vi "Dashboard Main Old.vi"() -> ()   [LabVIEW 2020]
uses:
  <vilib>/Rock Robotics/Network Tables/NT Read Numeric Array.vi
  <vilib>/Rock Robotics/Network Tables/NT Read String.vi
  <vilib>/Rock Robotics/Network Tables/NT Read Number.vi
  <vilib>/Rock Robotics/Network Tables/NT Read Boolean.vi
  <vilib>/Rock Robotics/Network Tables/NT Write Number.vi
  <vilib>/Rock Robotics/Network Tables/NT Write Boolean.vi
panel:
  out "Popcorn Engaged":bool
  out "Camera Image 5":T1(plugin-control)
  in  "Camera Settings Right":T2={"Frame Rate"=30, "Compression"=30, "Size"=1, "DB Camera Config"=FALSE} {"Frame Rate" scale=1.0..30.0; "Compression" scale=100.0..-1.0; "Size" items=["640x480", "320x240", "160x120"]}
  in  "Camera Name Right":string(combo)="No Camera Selection"
  out "Camera Perf":string
  in  "Camera Settings":T2={"Frame Rate"=30, "Compression"=30, "Size"=1, "DB Camera Config"=FALSE} {"Frame Rate" scale=1.0..30.0; "Compression" scale=100.0..-1.0; "Size" items=["640x480", "320x240", "160x120"]}
  in  "TCP":refnum<k5>
  out "Robot IP":string
  in  "Dashboard Tab":T3(tab)
  out "MotorChart R":cluster{"Numeric":dbl, "Numeric":dbl}(graph)
  out "MotorChart L":cluster{"Numeric":dbl, "Numeric":dbl}(graph)
  out "MotorSliders R":cluster{"MotorSlide1":dbl, "MotorSlide2":dbl} {"MotorSlide2" scale=-1.0..1.0 scale format="%#_2e"; "MotorSlide1" scale=-1.0..1.0 scale format="%#_2e"}
  out "MotorSliders L":cluster{"MotorSlide1":dbl, "MotorSlide2":dbl} {"MotorSlide2" scale=-1.0..1.0 scale format="%#_2e"; "MotorSlide1" scale=-1.0..1.0 scale format="%#_2e"}
  out "To infinity and beyond?":string
  out "Climb Override":bool
  out "Climbing Stages":sgl(slide) scale=0.0..10.0 scale format="%#_6p"
  out "Reverse":bool
  in  "ARE YOU READY TO RUMBLE":bool
  out "Drive Mode":string
  in  "Select Auto":string(combo)="Select Autonomous ..."
  out "NT Connection":bool
  out "JS1 Z":dbl(slide) scale=-1.0..1.0 scale format="%#_2e"
  out "JS1 Graph":cluster{"X":dbl, "Y":dbl}[](graph)
  out "JS1 Buttons":T4
  out "JS2 Z":dbl(slide) scale=-1.0..1.0 scale format="%#_2e"
  out "JS2 Graph":cluster{"X":dbl, "Y":dbl}[](graph)
  out "JS2 Buttons":T4
  out "Lidar":dbl(knob) scale=0.0..10.0
  out "Wall!":bool
  out "Mode":T5(ring)=enum."Auto Disabled"
  out "Camera Image Right":T1(plugin-control)
  out "Shooter Speed":cluster{"Shooter Demand":dbl, "Numeric":dbl}(graph)
  out "Shooter Speed":dbl
  in  "Shooter Demand":dbl
  in  "Dashboard Tab 2":T6(tab)
  out "Speed Chart Left":cluster{"Numeric":dbl, "Numeric":dbl}(graph)
  out "Speed Chart Right":cluster{"Numeric":dbl, "Numeric":dbl}(graph)
  in  "Boolean":bool
  out "Right Speed Demand":dbl
  out "Left Speed Demand":dbl
  out "Right Speed":dbl
  out "Left Speed":dbl
  out "Current Filter":T7={"Hue"={110.0, 142.0}, "Saturation"={0.0, 209.6394230769231}, "Value"={0.0, 105.16949152542372}} {"Value" scale=0.0..255.0; "Saturation" scale=0.0..255.0; "Hue" scale=0.0..255.0 scale format="%#_3g"}
  in  "New Filter":T7={"Hue"={110.0, 142.0}, "Saturation"={0.0, 209.6394230769231}, "Value"={0.0, 105.16949152542372}} {"Value" scale=0.0..255.0; "Saturation" scale=0.0..255.0; "Hue" scale=0.0..255.0 scale format="%#_3g"}
  out "Bananas Engaged":bool
  in  "DONUT PRESS":bool
  out "Bandwidth (Mbps)":dbl
  out "FPS":dbl
  in  "Update":bool
  in  "CheckList":i32[](listbox)
  out "Tree":string(tree)
  out "Camera Image":T1(plugin-control)
  out "Background":bool
  in  "Camera Name":string(combo)="No Camera Selection"
  # "HW"
  # "HW"
  # "Drive Motors"
  # "Joysticks"
  # "Front"
  # "Right"
  # "Left"
  # "Back"
  # "Right"
  # "Left"
  # "Speed D"
  # "Speed"
  # "DONUT PRESS"
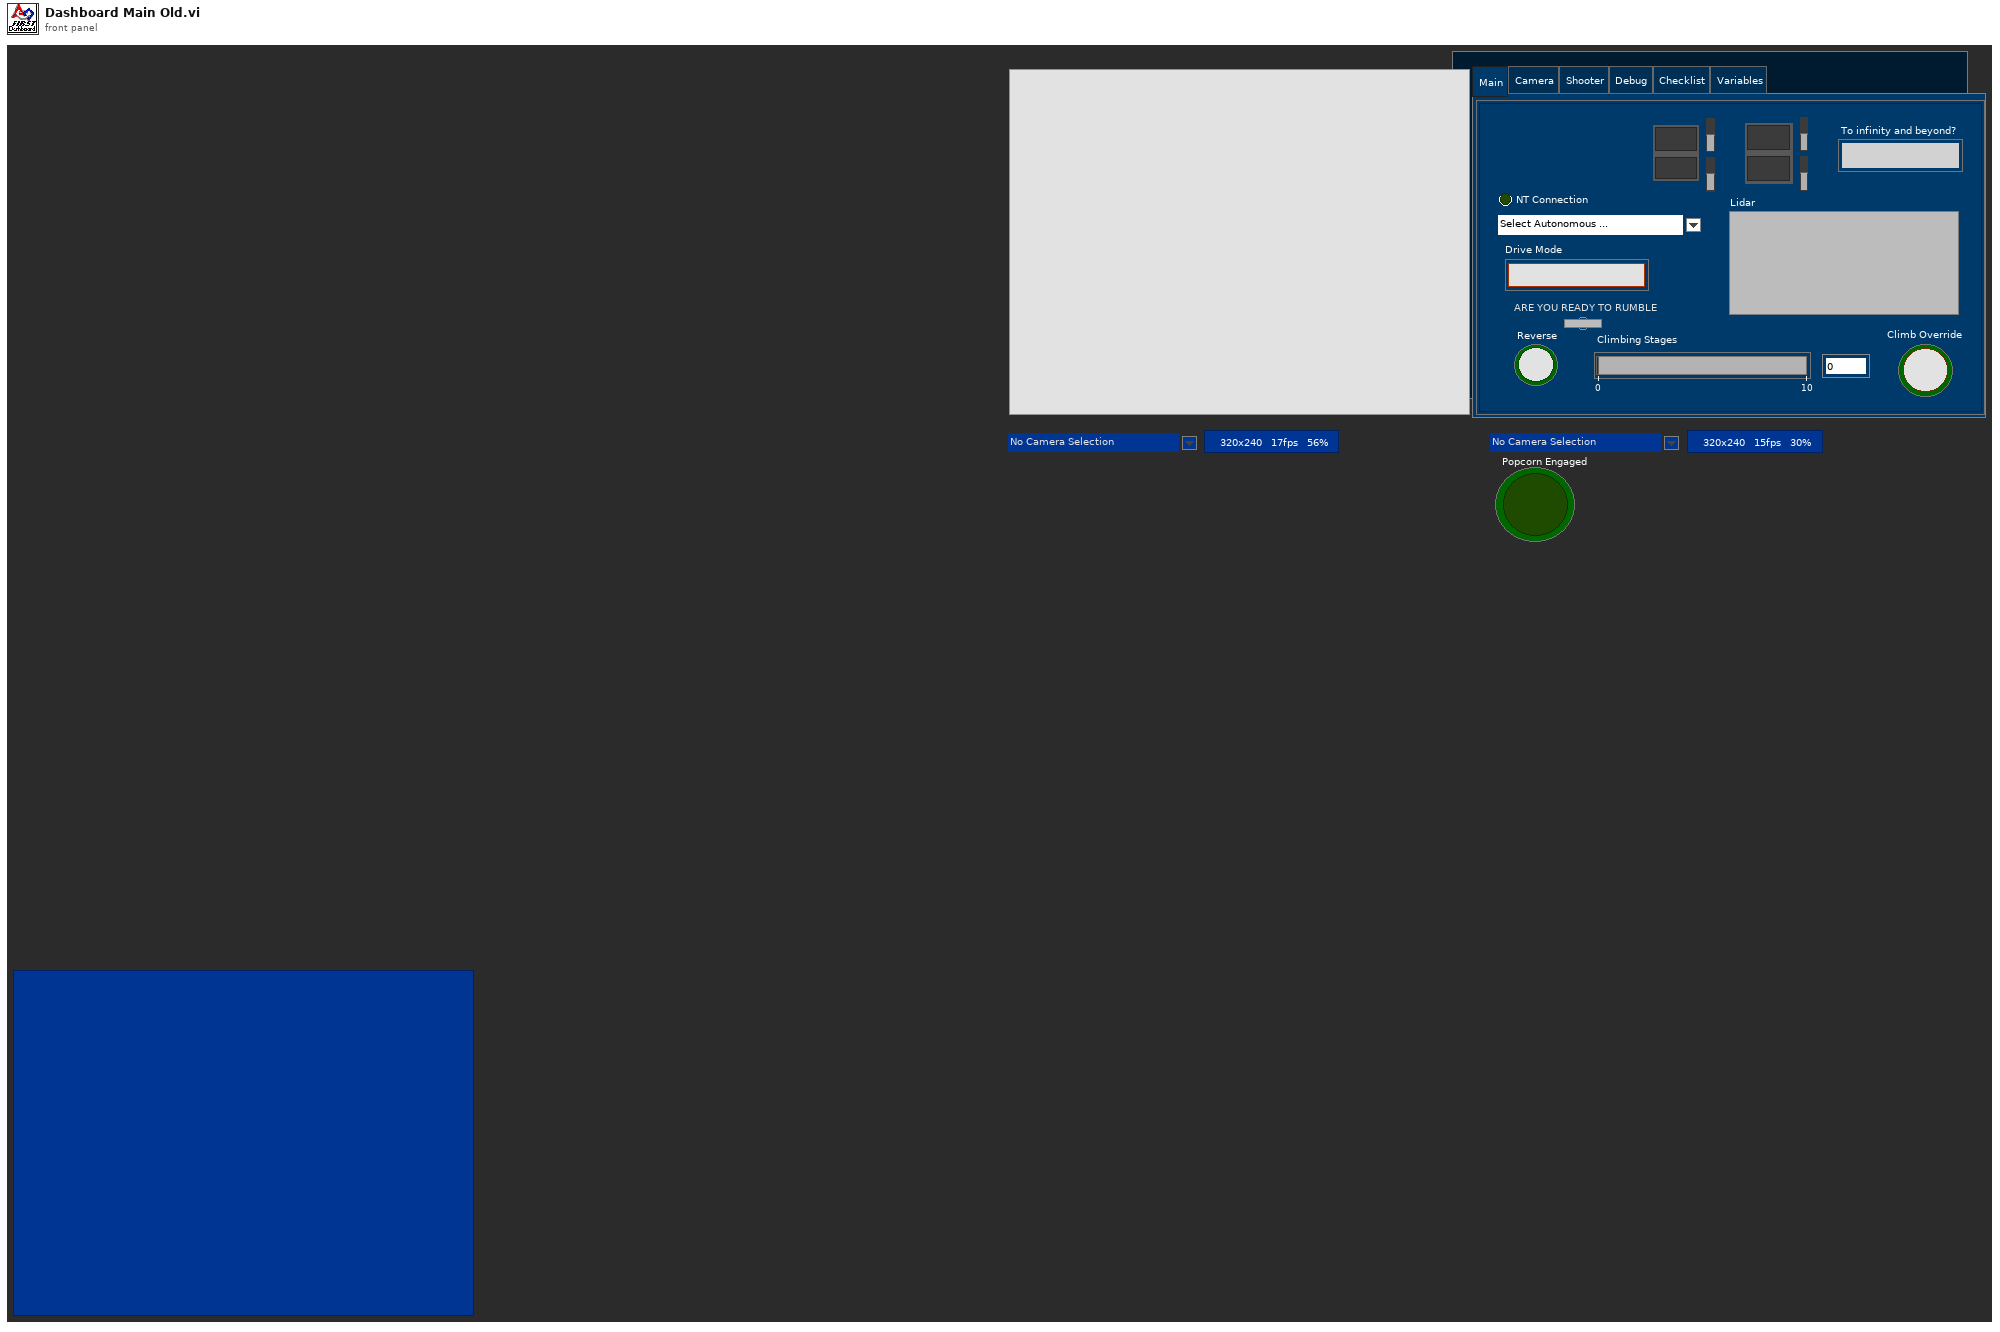
[diagram p1: front panel]
types:
  T1 = typedef "IMAQ Image.ctl" = refnum<image>
  T2 = cluster{"Frame Rate":i32, "Compression":i32, "Size":u16, "DB Camera Config":bool}
  T3 = enum32{"Main", "Camera", "Shooter", "Debug", "Checklist", "Variables"}
  T4 = cluster{bool, bool, bool, bool, bool, bool, bool, bool, bool, bool, bool, bool}
  T5 = enum8{"Tele-Op Disabled", "Tele-Op Enabled", "Auto Disabled", "Auto Enabled", "Test Disabled", "Test Enabled", "Disconnected", "No Code", "E-Stop"}
  T6 = enum32{"Drive Left", "Drive Right", "Table", "Camera", "Random"}
  T7 = cluster{"Hue":cluster{dbl, dbl}, "Saturation":cluster{dbl, dbl}, "Value":cluster{dbl, dbl}}
  T8 = typedef "Image Type" = u32
  T9 = cluster{"Save Path":path, "Interval (s)":dbl, "Keep":i32}
  T10 = cluster{"Camera Image":refnum<vi>, "Dashboard Tab":refnum<vi>, "Background":refnum<vi>, "Tree":refnum<vi>, "Camera Settings":refnum<vi>, "Camera Name":refnum<vi>, "Camera Perf":refnum<vi>}
  T11 = cluster{"Camera Name":string, "Camera File Name":string, "Saved DB Images Info":cluster{"Save Path":path, "Interval (s)":dbl, "Keep":i32}}
  T12 = cluster{cluster{dbl, dbl}, cluster{dbl, dbl}, cluster{dbl, dbl}}
  T13 = cluster{"Shift":bool, "Ctrl":bool, "Alt":bool, "Cmd":bool, "Opt":bool}
  T14 = cluster{"Global Rectangle":i32[], "Contours":cluster{"Contour Type":u32, "ROI Type":u32, "Points":i32[]}[]}
  T15 = cluster{"Camera Name Right":string, string, "Saved DB Images Info":cluster{"Save Path":path, "Interval (s)":dbl, "Keep":i32}}
  T16 = cluster{"Error Strings":string, "Disable Counts":cluster{u16, u16}, "Rail Faults":cluster{u16, u16, u16}, "Robot IP":string, "DB Mode":u8, "Event Info":cluster{"Name":string, "Type":u8, "Number":u16, "Replay":u8}}
  T17 = cluster{"Storage":cluster{"Disk Free":u64, "RAM Block":u32, "RAM free":u32}, "CPU Utilization":cluster{"CPU % ISR":sgl, "CPU % Time Crit":sgl, "CPU % Timed Str":sgl, "CPU % High":sgl, "CPU % Above":sgl, "CPU % Normal":sgl, "CPU % Low":sgl}, "CAN":cluster{"% Bus Utilization":sgl, "Bus Off Cnt":u32, "TX_FIFO Full Cnt":u32, "Receive Error Cnt":u8, "Transmit Error Cnt":u8}, "HID":cluster{"HID Outputs":u32, "Rumble Low":u16, "Rumble High":u16}[]}
  T18 = cluster{"Status bits":cluster{"Test Mode":bool, "Autonomous":bool, "Enabled":bool, "Code Start":bool, "Brownout":bool, "Reserved 2":bool, "Reserved 3":bool, "E-Stop":bool}, "Code Trace":cluster{"Disabled":bool, "TeleOp":bool, "Auto":bool, "Test":bool}, "Controller Type":enum16{"unknown", "cRIO", "roboRio"}, "Code?":enum16{"unknown", "noCode", "code"}, "Battery V":dbl}
  T19 = cluster{"Control Bits":cluster{"TestMode":bool, "Autonomous":bool, "Enabled":bool, "FMS Present":bool, bool, bool, bool, "E-Stop":bool}, "Team Station ":u8, "Countdown":sgl, "Joystick Values":cluster{"Axes":dbl[], "Buttons":bool[], "POVs":i16[]}[]}
  T20 = cluster{"Axes":dbl[], "Buttons":bool[], "POVs":i16[]}[]
  T21 = cluster{"Axes":dbl[], "Buttons":bool[], "POVs":i16[]}
  T22 = cluster{"Buttons[0]":bool, "Buttons[1]":bool, "Buttons[2]":bool, "Buttons[3]":bool, "Buttons[4]":bool, "Buttons[5]":bool, "Buttons[6]":bool, "Buttons[7]":bool, "Buttons[8]":bool, "Buttons[9]":bool, "Buttons[10]":bool, "Buttons[11]":bool}
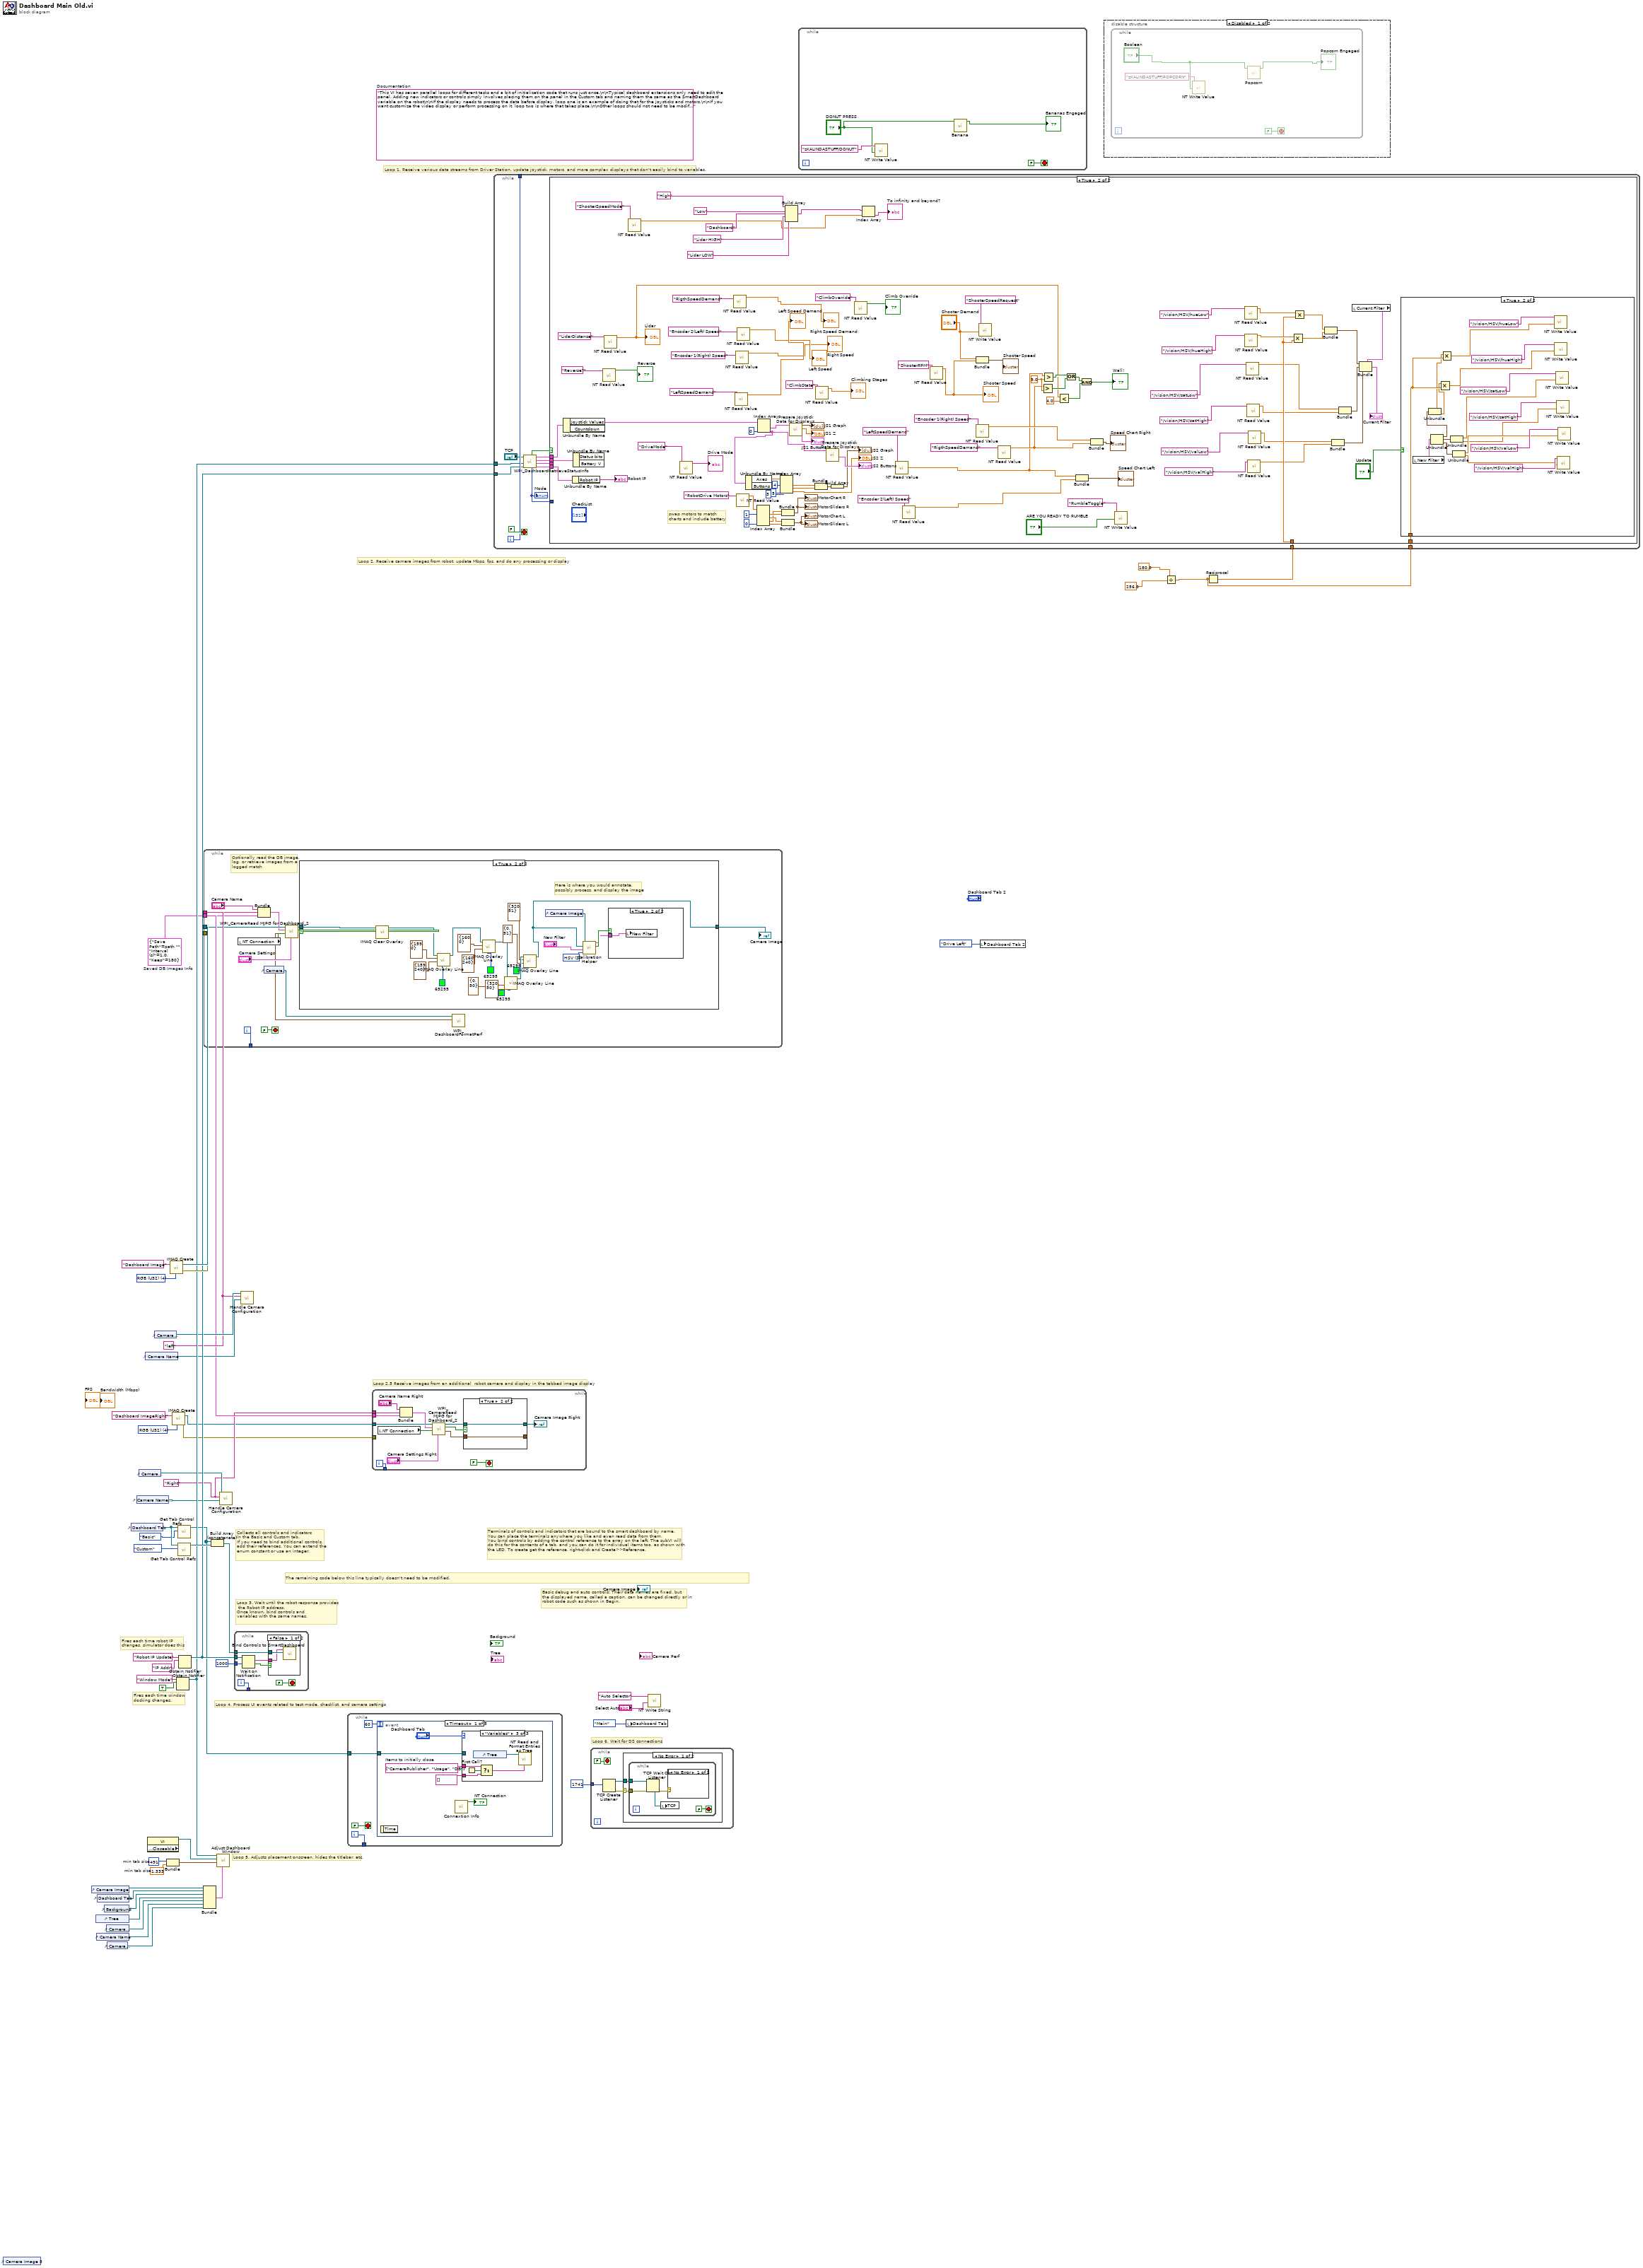
[diagram p0: block diagram]
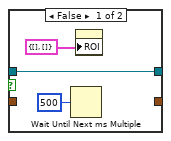
[diagram p3: hidden frame]
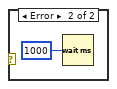
[diagram p4: hidden frame]
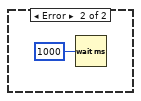
[diagram p5: hidden frame]
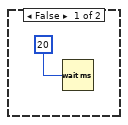
[diagram p6: hidden frame]
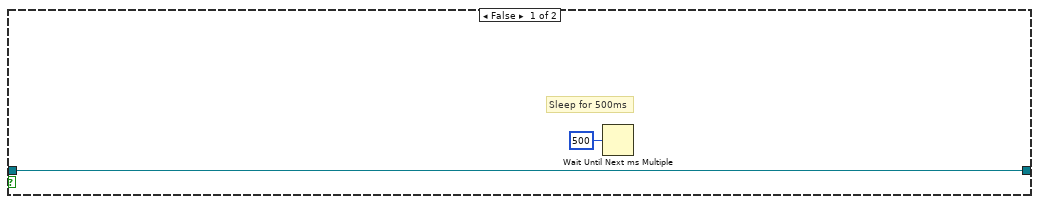
[diagram p9: hidden frame]
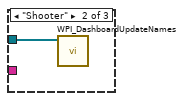
[diagram p12: hidden frame]
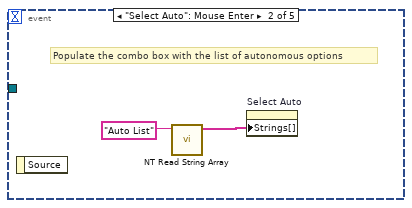
[diagram p13: hidden frame]
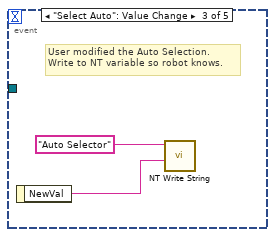
[diagram p14: hidden frame]
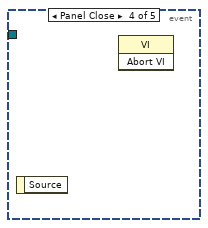
[diagram p15: hidden frame]
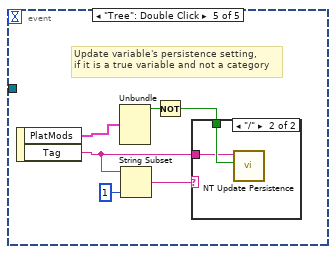
[diagram p16: hidden frame]
diagram:
  w8 = T8 4 items=["Grayscale (U8)", "Grayscale (I16)", "Grayscale (SGL)", "Complex (CSG)", "RGB (U32)", "HSL (U32)", "RGB (U64)"] ("Image Type")
  w10 = "Right"
  w14 = "left" ("Camera File Name")
  w13 = T9 {"Save Path"=path "", "Interval (s)"=1.0, "Keep"=180}  # Saved DB Images Info
  w34 = 491  # min tab size
  w33 = 1.333  # min tab size
  (unwired) "This VI has seven parallel loops for different tasks and a bit of initialization code that runs just once.\n\nTypical dashboard extensions only need to edit the panel. Adding new indicators or controls simply involves placing them on the panel in the Custom tab and naming them the same as the SmartDashboard variable on the robot\n\nIf the display needs to process the data before display, loop one is an example of doing that for the joysticks and motors.\n\nIf you want customize the video display or perform processing on it, loop two is where that takes place.\n\nOther loops should not need to be modified. They are pretty standard, and document the task they perform."  # Documentation
  w49 = T8 4 items=["Grayscale (U8)", "Grayscale (I16)", "Grayscale (SGL)", "Complex (CSG)", "RGB (U32)", "HSL (U32)", "RGB (U64)"] ("Image Type")
  # "Loop 2.5 Receive images from an additional  robot camera and display in the tabbed image display"
  # "Loop 6. Wait for DS connections"
  # "Basic debug and auto controls: Their data names are fixed, but\nthe displayed name, called a caption, can be changed directly or in\nrobot code such as shown in Begin."
  # "Fires each time robot IP\nchanges, simulator does this"
  # "Fires each time window\ndocking changes."
  # "Collects all controls and indicators\nin the Basic and Custom tab.\nIf you need to bind additional controls,\nadd their references. You can extend the\nenum constant or use an integer."
  # "The remaining code below this line typically doesn't need to be modified."
  # "Loop 4. Process UI events related to test mode, checklist, and camera settings"
  # "Terminals of controls and indicators that are bound to the smart dashboard by name.\nYou can place the terminals anywhere you like and even read data from them.\nYou bind controls by adding the control reference to the array on the left. The subVI will\ndo this for the contents of a tab, and you can do it for individual items too, as shown with\nthe LED. To create get the reference, right-click and Create>>Reference."
  # "Loop 3. Wait until the robot response provides\n the Robot IP address.\nOnce known, bind controls and\nvariables with the same names."
  # "Loop 5. Adjusts placement onscreen, hides the titlebar, etc."
  # "Loop 1. Receive various data streams from Driver Station, update joystick, motors, and more complex displays that don't easily bind to variables."
  # "Loop 2. Receive camera images from robot, update Mbps, fps, and do any processing or display"
  n1 = control-ref of="Camera Image 5"() -> ()  [unwired: 1 out]
  n2 = control-ref of="Camera Image"() -> (w36:refnum<vi>)
  n3 = control-ref of="Tree"() -> (w20:refnum<vi>)
  n4 = control-ref of="Camera Name"() -> (w18:refnum<vi>)
  n5 = control-ref of="Dashboard Tab"() -> (w35:refnum<vi>)
  n6 = control-ref of="Background"() -> (w31:refnum<vi>)
  n7 = control-ref of="Camera Settings"() -> (w19:refnum<vi>)
  n8 = control-ref of="Camera Perf"() -> (w17:refnum<vi>)
  n9 = control-ref of="Dashboard Tab"() -> (w39:refnum<vi>)
  n10 = control-ref of="Camera Name Right"() -> (w11:refnum<vi>)
  n11 = control-ref of="Camera Settings Right"() -> (w12:refnum<vi>)
  n12 = control-ref of="Camera Name"() -> (w24:refnum<vi>)
  n13 = property class="VI" props=["Front Panel.Closeable"]() -> (reference out=w40:refnum<vi>)  [unwired: 2 in, 2 out]
  n14 = control-ref of="Camera Settings"() -> (w25:refnum<vi>)
  n15 = Bundle("min tab size"=w34, "min tab size"=w33) -> (w32:cluster{"min tab size":i32, "min tab size":dbl})  [unwired: 1 in]
  n16 = call "IMAQ Create"("Image Name"="Dashboard Image", "Image Type"=w49) -> ("New Image"=w47:T1, "error out"=w46:errorcluster)  [unwired: 2 in, 1 out]
  n17 = call "IMAQ Create"("Image Name"="Dashboard ImageRight", "Image Type"=w8) -> ("New Image"=w7:T1, "error out"=w6:errorcluster)  [unwired: 2 in, 1 out]
  n18 = Obtain Notifier(name (unnamed)="Window Mode", notification data type=TRUE) -> (notifier out=w28:refnum<notifier>)  [unwired: 2 in, 2 out]
  n19 = call <vilib>:"Get Tab Control Refs.vi"("Page Index"=enum32{"Drive", "Basic", "Custom", "Variables"}."Basic" ("Dashboard Tab"), "TabControl in"=w39) -> ("ControlsOnPage"=w23:refnum<vi>[])  [unwired: 9 in]
  n20 = call <vilib>:"Get Tab Control Refs.vi"("Page Index"=enum32{"Drive", "Basic", "Custom", "Variables"}."Custom" ("Dashboard Tab"), "TabControl in"=w39) -> ("ControlsOnPage"=w38:refnum<vi>[])  [unwired: 9 in]
  n21 = Obtain Notifier(name (unnamed)="Robot IP Update", notification data type="IP Addr" ("name (unnamed)")) -> (notifier out=w29:refnum<notifier>)  [unwired: 2 in, 2 out]
  n22 = Bundle("Camera Image"=w36, "Dashboard Tab"=w35, "Background"=w31, "Tree"=w20, "Camera Settings"=w19, "Camera Name"=w18, "Camera Perf"=w17) -> (w30:T10)  [unwired: 1 in]
  n23 = while {
    tunnel: w47 -> [w61]
    tunnel: w46 -> [_]
    tunnel: [w62] -> _
    tunnel: w13 -> [w55]
    tunnel: w14 -> [w53]
    i -> [w62]
    stop <- FALSE stop-if-true
    # "Optionally read the DB image,\nlog, or retrieve images from a\nlogged match"
    n24 = local read "NT Connection"() -> (w56:bool)
    n25 = Bundle("Camera Name"="Camera Name", "Camera File Name"=w53, "Saved DB Images Info"=w55) -> (w54:T11)  [unwired: 1 in]
    n26 = control-ref of="Camera Perf"() -> (w51:refnum<vi>)
    n27 = call <vilib>:"WPI_CameraRead MJPG for Dashboard_2.vi"("Camera Settings"="Camera Settings", "NT Connection"=w56, "Capture Info"=w54, "Image in"=w61) -> ("perf info"=w52:cluster{"Bandwidth (Mbps)":dbl, "fps":dbl}, "Active"=w59:bool, "Image\\ out"=w60:T1)  [unwired: 5 in]
    n28 = case shown="True" w59 {
      tunnel: w60 -> [w64 w88]
      tunnel: [w64 w72] -> w57
      frame False {
        # "Sleep for 500ms"
        n29 = Wait Until Next ms Multiple(millisecond multiple=u32 500) -> ()  [unwired: 1 out]
      }
      frame True {
        w84 = u16 2 items=["RGB", "HSL", "HSV", "HSI", "CIE L*a*b*", "CIE XYZ"] ("Color Mode")
        # "Here is where you would annotate,\npossibly process, and display the image"
        n30 = call "IMAQ Clear Overlay"("Image"=w88) -> ("Image Out"=w82:T1)  [unwired: 2 in, 8 out]
        n31 = call "IMAQ Overlay Line"("Color"=u32 65295, "End Point"=cluster{"X":i32, "Y":i32} {"X"=159, "Y"=240}, "Start Point"=cluster{"X":i32, "Y":i32} {"X"=159, "Y"=0}, "Image"=w82) -> ("Image Out"=w78:T1)  [unwired: 6 in, 1 out]
        n32 = call "IMAQ Overlay Line"("Color"=u32 65295, "End Point"=cluster{"X":i32, "Y":i32} {"X"=160, "Y"=240}, "Start Point"=cluster{"X":i32, "Y":i32} {"X"=160, "Y"=0}, "Image"=w78) -> ("Image Out"=w73:T1)  [unwired: 6 in, 1 out]
        n33 = call "IMAQ Overlay Line"("Color"=u32 65295, "End Point"=cluster{"X":i32, "Y":i32} {"X"=0, "Y"=50}, "Start Point"=cluster{"X":i32, "Y":i32} {"X"=320, "Y"=50}, "Image"=w73) -> ("Image Out"=w74:T1)  [unwired: 6 in, 1 out]
        n34 = call "IMAQ Overlay Line"("Color"=u32 65295, "End Point"=cluster{"X":i32, "Y":i32} {"X"=0, "Y"=51}, "Start Point"=cluster{"X":i32, "Y":i32} {"X"=320, "Y"=51}, "Image"=w74) -> ("Image Out"=w72:T1)  [unwired: 6 in, 1 out]
        n35 = control-ref of="Camera Image"() -> (w83:refnum<vi>)
        n36 = call "Calibration Helper.vi"("Color Mode"=w84, "Color Components"="New Filter", "Image"=w72, "Image Ctl Refnum"=w83) -> ("Changed"=w86:bool, "output color"=w85:T12)  [unwired: 6 in]
        n37 = case shown="True" w86 {
          tunnel: w85 -> [_ w89]
          frame False {
          }
          frame True {
            n38 = local write "New Filter"(w89) -> ()
          }
        }
      }
    }
    "Camera Image" <- w57
    n39 = call <vilib>:"WPI_DashboardFormatPerf.vi"("Performance"=w52, "String in"=w51) -> ()  [unwired: 10 in]
  }
  n40 = Build Array (concatenate)(w23, w38) -> (w37:refnum<vi>[])
  n41 = call "Adjust Dashboard Window.vi"("Sizing Refnums"=w30, "Size Constraints"=w32, "VI"=w40, "WIn Mode"=w28) -> ()  [unwired: 8 in]
  n42 = call "Handle Camera Configuration.vi"("CameraNameRef"=w11, "Display Name"=w10, "ClusterRef"=w12) -> ()  [unwired: 9 in]
  n43 = while {
    tunnel: w37 -> [w96]
    tunnel: w29 -> [w94]
    tunnel: [w92] -> _
    tunnel: u32 1000 ("milliseconds to wait") -> [w91]
    i -> [w92]
    stop <- FALSE stop-if-true
    n44 = Wait on Notification(notifier=w94, timeout in ms (-1)=w91) -> (notification=w93:string, timed out?=w90:bool)  [unwired: 2 in, 2 out]
    n45 = case shown="False" w90 {
      tunnel: w96 -> [w98 _]
      tunnel: w93 -> [w97 _]
      frame False {
        n46 = call <vilib>:"Bind Controls to SmartDashboard.vi"("Bound Control Refs"=w98, "Server IP Address"=w97) -> ()  [unwired: 10 in]
      }
      frame True {
      }
    }
  }
  n47 = call "Handle Camera Configuration.vi"("CameraNameRef"=w24, "Display Name"=w14, "ClusterRef"=w25) -> ()  [unwired: 9 in]
  n48 = while {
    tunnel: [w100] -> _
    tunnel: w23 -> [w99]
    i -> [w100]
    stop <- FALSE stop-if-true
    n49 = event shown="[0] Timeout" {
      selector: _ -> [_ _ _ _ _]
      dyn-events: _ -> [_ _ _ _ _]
      timeout: u32 60 ("milliseconds to wait") -> [_ _ _ _ _]
      tunnel: w99 -> [w105 _ _ _ _]
      event Timeout {
        w104 = string[] ["CameraPublisher", "Usage", "DB"]  # Items to initially close
        n50 = event-data() -> ()  [unwired: 1 in, 1 out]
        n51 = call <vilib>:"Connextion Info.vi"() -> ("Connected"=→"NT Connection":bool)  [unwired: 10 in, 1 out]
        n52 = case shown="\"Variables\"" "Dashboard Tab" {
          tunnel: w105 -> [_ w108 _]
          tunnel: w104 -> [_ _ w111]
          tunnel: string[] [] -> [_ _ w110]
          frame "Debug", Default {
          }
          frame "Shooter" {
            n53 = call <vilib>:"WPI_DashboardUpdateNames.vi"("Controls on Tab"=w108) -> ()  [unwired: 11 in]
          }
          frame "Variables" {
            n54 = First Call?() -> (First Call?: T/F=w112:bool)
            n55 = control-ref of="Tree"() -> (w113:refnum<vi>)
            n56 = Select(t=w111, s=w112, f=w110) -> (s? t:f=w109:string[])
            n57 = call <vilib>:"NT Read and Format Entries as Tree.vi"("Tags to  Close"=w109, "Tree Refnum"=w113) -> ()  [unwired: 8 in, 2 out]
          }
        }
      }
      event "Select Auto": Mouse Enter {
        # "Populate the combo box with the list of autonomous options"
        n58 = event-data() -> ()  [unwired: 1 in, 1 out]
        n59 = call <vilib>:"NT Read String Array.vi"("Name"="Auto List") -> ("String Array"=w114:string[])  [unwired: 9 in, 1 out]
        n60 = property on="Select Auto" class="CmbBox"("Strings[]"=w114) -> ()  [unwired: 2 in, 2 out]
      }
      event "Select Auto": Value Change {
        # "User modified the Auto Selection.\nWrite to NT variable so robot knows."
        n61 = event-data() -> ("NewVal"=w116:string)  [unwired: 1 in]
        n62 = call <vilib>:"NT Write String.vi"("String"=w116, "Name"="Auto Selector") -> ()  [unwired: 9 in, 1 out]
      }
      event Panel Close {
        n63 = event-data() -> ()  [unwired: 1 in, 1 out]
        n64 = invoke class="VI" method="Abort VI"() -> ()  [unwired: 3 in, 3 out]
      }
      event "Tree": Double Click {
        # "Update variable's persistence setting,\nif it is a true variable and not a category"
        n65 = event-data() -> ("PlatMods"=w119:T13, "Tag"=w118:string)  [unwired: 1 in]
        n66 = Unbundle(w119) -> ("Shift"=w123:bool)  [unwired: 4 out]
        n67 = String Subset(string=w118, length (rest)=1 ("length (rest)")) -> (substring=w120:string)  [unwired: 1 in]
        n68 = Not(x=w123) -> (.not. x?=w122:bool)
        n69 = case shown="\"/\"" w120 {
          tunnel: w122 -> [_ w125]
          tunnel: w118 -> [_ w124]
          frame Default {
          }
          frame "/" {
            n70 = call <vilib>:"NT Update Persistence.vi"("Persistence"=w125, "Name"=w124) -> ()  [unwired: 9 in, 1 out]
          }
        }
      }
    }
  }
  n71 = while {
    tunnel: w7 -> [w138]
    tunnel: [w134] -> _
    tunnel: w13 -> [w130]
    tunnel: w10 -> [w127]
    tunnel: w6 -> [_]
    i -> [w134]
    stop <- FALSE stop-if-true
    n72 = local read "NT Connection"() -> (w131:bool)
    n73 = Bundle("Camera Name Right"="Camera Name Right", w127, "Saved DB Images Info"=w130) -> (w129:T15)  [unwired: 1 in]
    n74 = call <vilib>:"WPI_CameraRead MJPG for Dashboard_2.vi"("Camera Settings"="Camera Settings Right", "NT Connection"=w131, "Capture Info"=w129, "Image in"=w138) -> ("perf info"=w126:cluster{"Bandwidth (Mbps)":dbl, "fps":dbl}, "Active"=w133:bool, "Image\\ out"=w136:T1)  [unwired: 5 in]
    n75 = case shown="True" w133 {
      tunnel: w136 -> [w140 w143]
      tunnel: [w140 w143] -> w132
      tunnel: [_ w142] -> _
      tunnel: w126 -> [_ w142]
      frame False {
        n76 = Wait Until Next ms Multiple(millisecond multiple=u32 500) -> ()  [unwired: 1 out]
        n77 = property on="Camera Image Right" class="ImageControl"("ROI"=T14 {"Global Rectangle"=[], "Contours"=[]}) -> ()  [unwired: 2 in, 2 out]
      }
      frame True {
      }
    }
    "Camera Image Right" <- w132
  }
  n78 = while {
    tunnel: u16 1741 ("timeout ms (25000)") -> [w145]
    stop <- FALSE stop-if-true
    n79 = TCP Create Listener(10:w145) -> (0:w144:errorcluster, 3:w146:refnum<k5>)  [unwired: 4 in, 1 out]
    n80 = case shown="No Error" w144 {
      selector: w144 -> [w148 _]
      tunnel: w146 -> [w149 _]
      frame No Error {
        n81 = while {
          tunnel: w149 -> [w152]
          tunnel: w148 -> [w151]
          stop <- FALSE stop-if-true
          n82 = TCP Wait On Listener(8:w151, 11:w152) -> (0:w153:errorcluster, 4:w154:refnum<k5>)  [unwired: 2 in, 3 out]
          n83 = local write "TCP"(w154) -> ()
          n84 = case shown="No Error" w153 {
            frame No Error {
            }
            frame Error {
              n85 = Wait (ms)(milliseconds to wait=u32 1000) -> ()  [unwired: 1 out]
            }
          }
        }
      }
      frame Error {
        n86 = Wait (ms)(milliseconds to wait=u32 1000) -> ()  [unwired: 1 out]
      }
    }
  }
  n87 = local write "Dashboard Tab"(T3."Main" ("Dashboard Tab")) -> ()
  n88 = call <vilib>:"NT Write String.vi"("String"="Select Auto", "Name"="Auto Selector") -> ()  [unwired: 9 in, 1 out]
  n89 = while {
    stop <- FALSE stop-if-true
    n90 = call-poly <vilib>:"NT Write Value.vi"("Boolean"="DONUT PRESS", "Name"="zKALINDASTUFF/DONUT") -> ()  [unwired: 9 in, 1 out]
    n91 = call "Banana.vi"("Boolean"="DONUT PRESS") -> ("Boolean 2"=→"Bananas Engaged":bool)  [unwired: 10 in]
  }
  n92 = local write "Dashboard Tab 2"(T6."Drive Left" ("Dashboard Tab")) -> ()
  n93 = disable-structure shown="Disabled" {
    frame Disabled {
      n94 = while {
        stop <- FALSE stop-if-true
        n95 = call-poly <vilib>:"NT Write Value.vi"("Boolean"="Boolean", "Name"="zKALINDASTUFF/POPCORN") -> ()  [unwired: 9 in, 1 out]
        n96 = call "Popcorn.vi"("Boolean"="Boolean") -> ("Boolean 2"=→"Popcorn Engaged":bool)  [unwired: 10 in]
      }
    }
    frame Enabled {
    }
  }
  n97 = Divide(x=180.0, y=256.0) -> (x/y=w1:dbl)
  n98 = Reciprocal(x=w1) -> (1/x=w2:dbl)
  n99 = while {
    tunnel: [w176] -> _
    tunnel: w29 -> [w170]
    tunnel: w28 -> [w167]
    tunnel: w2 -> [w166]
    tunnel: w1 -> [w165]
    i -> [w176]
    stop <- FALSE stop-if-true
    n100 = call <vilib>:"WPI_DashboardRetrieveStatusInfo.vi"("Binding Refnum"=w170, "Window Mode Notifier"=w167, "TCP Cnx"="TCP") -> ("Power and Errors"=w171:T16, "Robot Metrics"=w174:T17, "Status Info"=w175:T18, "Control Info"=w172:T19, "Robot Mode"=w169:T5, "Process?"=w173:bool)  [unwired: 3 in]
    "Mode" <- w169
    n101 = case shown="True" w173 {
      tunnel: w175 -> [_ w282]
      tunnel: w174 -> [_ _]
      tunnel: w172 -> [_ w281]
      tunnel: w171 -> [_ w280]
      tunnel: w169 -> [_ _]
      tunnel: w166 -> [_ w227]
      tunnel: w165 -> [_ w216]
      frame False {
        n102 = Wait (ms)(milliseconds to wait=u32 20) -> ()  [unwired: 1 out]
      }
      frame True {
        w183 = 9.0 ("y")
        # "swap motors to match\ncharts and include battery"
        n103 = Unbundle By Name(w281) -> ("Joystick Values"=w271:T20)  [unwired: 1 out]
        n104 = Unbundle By Name(w280) -> ("Robot IP"=→"Robot IP":string)
        n105 = Unbundle By Name(w282) -> ()  [unwired: 2 out]
        n106 = call-poly <vilib>:"NT Read Value.vi"("Name"="Reverse?") -> ("Boolean"=→"Reverse":bool)  [unwired: 9 in, 1 out]
        n107 = call-poly <vilib>:"NT Read Value.vi"("Name"="LidarDistance") -> ("Numeric"=w179:dbl)  [unwired: 9 in, 1 out]
        "Lidar" <- w179
        n108 = call-poly <vilib>:"NT Read Value.vi"("Name"="ShooterSpeedMode") -> ("Numeric"=w190:dbl)  [unwired: 9 in, 1 out]
        n109 = call-poly <vilib>:"NT Read Value.vi"("Name"="DriveMode") -> ("String"=→"Drive Mode":string)  [unwired: 9 in, 1 out]
        n110 = call-poly <vilib>:"NT Read Value.vi"("Name"="RigthSpeedDemand") -> ("Numeric"=→"Right Speed Demand":dbl)  [unwired: 9 in, 1 out]
        n111 = call-poly <vilib>:"NT Read Value.vi"("Name"="LeftSpeedDemand") -> ("Numeric"=→"Left Speed Demand":dbl)  [unwired: 9 in, 1 out]
        n112 = call-poly <vilib>:"NT Read Value.vi"("Name"="Encoder 1(Right) Speed") -> ("Numeric"=→"Right Speed":dbl)  [unwired: 9 in, 1 out]
        n113 = call-poly <vilib>:"NT Read Value.vi"("Name"="RobotDrive Motors") -> ("Numeric Array"=w264:dbl[])  [unwired: 9 in, 1 out]
        n114 = call-poly <vilib>:"NT Read Value.vi"("Name"="Encoder 2(Left) Speed") -> ("Numeric"=→"Left Speed":dbl)  [unwired: 9 in, 1 out]
        n115 = Index Array(array=w264, index #1=1, index #4=0) -> (element #1=w275:dbl, element #2=w276:dbl, element #3=w274:dbl, element #4=w279:dbl)  [unwired: 2 in]
        n116 = Index Array(array=w271, index #2=0 ("index")) -> (element #1=w270:T21, element #2=w203:T21)  [unwired: 1 in]
        n117 = Unbundle By Name(w203) -> ("Axes"=w207:dbl[])  [unwired: 1 out]
        n118 = Index Array(array=w207, index #1=4 ("index"), index #2=5 ("index"), index #3=3 ("index")) -> (element #1=w205:dbl, element #2=w204:dbl, element #3=→"JS2 Z":dbl)
        n119 = Bundle("Numeric"=w274, "Numeric"=w275) -> (→"MotorChart R" →"MotorSliders R":cluster{"Numeric":dbl, "Numeric":dbl})  [unwired: 1 in]
        n120 = Bundle("Numeric"=w276, "Numeric"=w279) -> (→"MotorChart L" →"MotorSliders L":cluster{"Numeric":dbl, "Numeric":dbl})  [unwired: 1 in]
        n121 = Build Array("High", "Low", "Dashboard", "Lidar HIGH", "Lidar LOW") -> (w191:string[])
        n122 = call "Prepare Joystick Data for Displays.vi"("Joystick Values"=w270) -> ("Buttons"=→"JS1 Buttons":T22, "Z Axis"=→"JS1 Z":dbl, "Cartesian Data"=→"JS1 Graph":cluster{"X axis":dbl, "X axis":dbl}[])  [unwired: 8 in]
        n123 = Bundle("X axis"=w205, "X axis"=w204) -> (w206:cluster{"X axis":dbl, "X axis":dbl})  [unwired: 1 in]
        n124 = call-poly <vilib>:"NT Read Value.vi"("Name"="ClimbState") -> ("Numeric"=→"Climbing Stages":dbl)  [unwired: 9 in, 1 out]
        n125 = call "Prepare Joystick Data for Displays.vi"("Joystick Values"=w203) -> ("Buttons"=→"JS2 Buttons":T22)  [unwired: 8 in, 2 out]
        n126 = Build Array(w206) -> (→"JS2 Graph":cluster{"X axis":dbl, "X axis":dbl}[])
        n127 = call-poly <vilib>:"NT Read Value.vi"("Name"="ClimbOverride") -> ("Boolean"=→"Climb Override":bool)  [unwired: 9 in, 1 out]
        n128 = Index Array(array=w191, index=w190) -> (element=→"To infinity and beyond?":string)
        n129 = call-poly <vilib>:"NT Read Value.vi"("Name"="LeftSpeedDemand") -> ("Numeric"=w181:dbl)  [unwired: 9 in, 1 out]
        n130 = call-poly <vilib>:"NT Read Value.vi"("Name"="Encoder 2(Left) Speed") -> ("Numeric"=w256:dbl)  [unwired: 9 in, 1 out]
        n131 = call-poly <vilib>:"NT Read Value.vi"("Name"="ShooterRPM") -> ("Numeric"=w237:dbl)  [unwired: 9 in, 1 out]
        "Shooter Speed" <- w237
        n132 = Bundle("Shooter Demand"="Shooter Demand", "Numeric"=w237) -> (→"Shooter Speed":cluster{"Shooter Demand":dbl, "Numeric":dbl})  [unwired: 1 in]
        n133 = call-poly <vilib>:"NT Read Value.vi"("Name"="Encoder 1(Right) Speed") -> ("Numeric"=w255:dbl)  [unwired: 9 in, 1 out]
        n134 = call-poly <vilib>:"NT Write Value.vi"("Numeric"="Shooter Demand", "Name"="ShooterSpeedRequest") -> ()  [unwired: 9 in, 1 out]
        n135 = call-poly <vilib>:"NT Read Value.vi"("Name"="RigthSpeedDemand") -> ("Numeric"=w182:dbl)  [unwired: 9 in, 1 out]
        n136 = Greater?(x=w182, y=w183) -> (0:w187:bool)
        n137 = Greater?(x=w181, y=w183) -> (0:w188:bool)
        n138 = Less?(x=w179, y=4.0) -> (x < y?=w186:bool)
        n139 = Or(x=w188, y=w187) -> (x .or. y?=w185:bool)
        n140 = Bundle("Numeric"=w181, "Numeric"=w256) -> (→"Speed Chart Left":cluster{"Numeric":dbl, "Numeric":dbl})  [unwired: 1 in]
        n141 = And(x=w185, y=w186) -> (x .and. y?=→"Wall!":bool)
        n142 = Bundle("Numeric"=w255, "Numeric"=w182) -> (→"Speed Chart Right":cluster{"Numeric":dbl, "Numeric":dbl})  [unwired: 1 in]
        n143 = call-poly <vilib>:"NT Write Value.vi"("Boolean"="ARE YOU READY TO RUMBLE", "Name"="RumbleToggle") -> ()  [unwired: 9 in, 1 out]
        n144 = call-poly <vilib>:"NT Read Value.vi"("Name"="/vision/HSV/hueLow") -> ("Numeric"=w229:dbl)  [unwired: 9 in, 1 out]
        n145 = call-poly <vilib>:"NT Read Value.vi"("Name"="/vision/HSV/hueHigh") -> ("Numeric"=w228:dbl)  [unwired: 9 in, 1 out]
        n146 = call-poly <vilib>:"NT Read Value.vi"("Name"="/vision/HSV/satLow") -> ("Numeric"=w224:dbl)  [unwired: 9 in, 1 out]
        n147 = call-poly <vilib>:"NT Read Value.vi"("Name"="/vision/HSV/satHigh") -> ("Numeric"=w223:dbl)  [unwired: 9 in, 1 out]
        n148 = call-poly <vilib>:"NT Read Value.vi"("Name"="/vision/HSV/valHigh") -> ("Numeric"=w221:dbl)  [unwired: 9 in, 1 out]
        n149 = call-poly <vilib>:"NT Read Value.vi"("Name"="/vision/HSV/valLow") -> ("Numeric"=w222:dbl)  [unwired: 9 in, 1 out]
        n150 = Multiply(x=w228, y=w227) -> (x*y=w225:dbl)
        n151 = Multiply(x=w229, y=w227) -> (x*y=w226:dbl)
        n152 = Bundle(w226, w225) -> (w220:cluster{dbl, dbl})  [unwired: 1 in]
        n153 = Bundle("Numeric"=w222, "Numeric"=w221) -> (w218:cluster{"Numeric":dbl, "Numeric":dbl})  [unwired: 1 in]
        n154 = Bundle("Numeric"=w224, "Numeric"=w223) -> (w219:cluster{"Numeric":dbl, "Numeric":dbl})  [unwired: 1 in]
        n155 = local read "Current Filter"() -> (w215:T7)
        n156 = Bundle(cluster=w215, "Hue"=w220, "Saturation"=w219, "Value"=w218) -> (→"Current Filter":T7)
        n157 = case shown="True" "Update" {
          tunnel: w216 -> [_ w294]
          frame False {
          }
          frame True {
            n158 = local read "New Filter"() -> (w295:T7)
            n159 = Unbundle(w295) -> ("Hue"=w293:cluster{dbl, dbl}, "Saturation"=w288:cluster{dbl, dbl}, "Value"=w287:cluster{dbl, dbl})
            n160 = Unbundle(w293) -> (w292:dbl, w291:dbl)
            n161 = Multiply(x=w291, y=w294) -> (x*y=w289:dbl)
            n162 = Multiply(x=w292, y=w294) -> (x*y=w290:dbl)
            n163 = Unbundle(w288) -> (w284:dbl, w283:dbl)
            n164 = Unbundle(w287) -> (w286:dbl, w285:dbl)
            n165 = call-poly <vilib>:"NT Write Value.vi"("Numeric"=w290, "Name"="/vision/HSV/hueLow") -> ()  [unwired: 9 in, 1 out]
            n166 = call-poly <vilib>:"NT Write Value.vi"("Numeric"=w289, "Name"="/vision/HSV/hueHigh") -> ()  [unwired: 9 in, 1 out]
            n167 = call-poly <vilib>:"NT Write Value.vi"("Numeric"=w284, "Name"="/vision/HSV/satLow") -> ()  [unwired: 9 in, 1 out]
            n168 = call-poly <vilib>:"NT Write Value.vi"("Numeric"=w283, "Name"="/vision/HSV/satHigh") -> ()  [unwired: 9 in, 1 out]
            n169 = call-poly <vilib>:"NT Write Value.vi"("Numeric"=w285, "Name"="/vision/HSV/valHigh") -> ()  [unwired: 9 in, 1 out]
            n170 = call-poly <vilib>:"NT Write Value.vi"("Numeric"=w286, "Name"="/vision/HSV/valLow") -> ()  [unwired: 9 in, 1 out]
          }
        }
      }
    }
  }
